vi "Command Create (0 parameters).vi"(9 "Command Mode":enum16{"Write", "Read"}(ring), 10 "Command Type":T1(ring), 11 "Command Name":string) -> (2 "Command":string)   [LabVIEW 2017, in "Roboteq Controller KBL1xxx.lvlib"]
uses:
  <instrlib>/Roboteq Controller KBL1xxx/Roboteq Controller KBL1xxx.lvlib
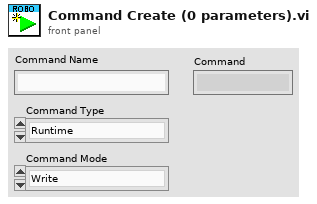
[diagram p1: front panel]
types:
  T1 = enum16{"Runtime", "Configuration", "Maintenance"}
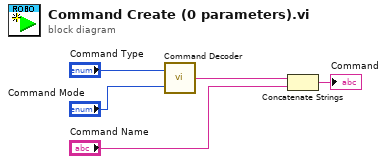
[diagram p0: block diagram]
diagram:
  n1 = call <instrlib>:"Command Decoder.vi"("Command Mode"="Command Mode", "Command Type"="Command Type") -> ("Start symbol"=w3:string)
  n2 = Concatenate Strings(w3, "Command Name") -> (→"Command":string)
